vi "Get IP Name.vi"(8 "error in (no error)":errorcluster, 11 "Engine Simulation IP in":refnum<class "Engine Simulation IP.lvclass">) -> (0 "error out":errorcluster, 2 "Name":string, 3 "Engine Simulation IP out":refnum<class "Engine Simulation IP.lvclass">)   [LabVIEW 2013, in "Engine Simulation IP.lvclass"]
uses:
  Engine Simulation IP.lvclass
  Engine Simulation IP.lvclass/Engine Simulation IP.ctl
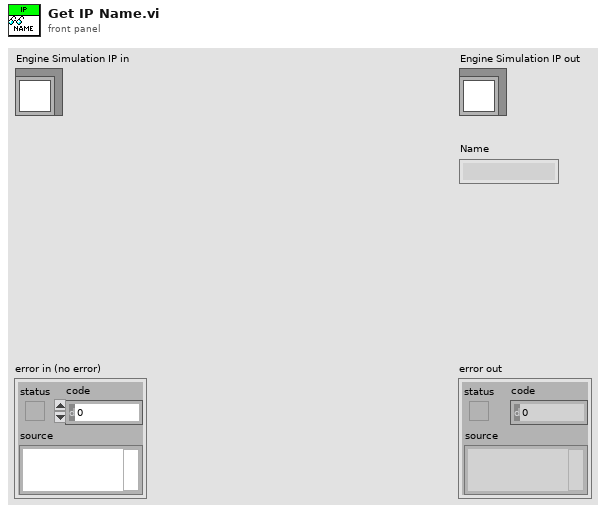
[diagram p1: front panel]
types:
  T1 = typedef "Engine Simulation IP.lvclass/IP class private data.ctl" = cluster{"Name":string, "EST version":T2, "session":refnum<class "Engine Simulation Session.lvclass">}
  T2 = typedef "Engine Simulation Session.lvclass/Bitfile Major Version.ctl" = enum16{"1.0", "1.1", "1.2", "1.3"}
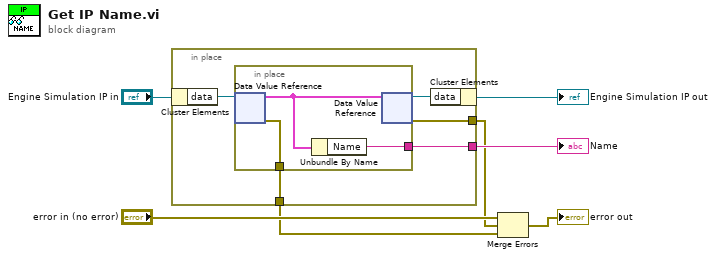
[diagram p0: block diagram]
diagram:
  n1 = in-place {
    in-place-border: [w12] -> w6
    in-place-border: [w9] -> w2
    in-place-border: [w8] -> w1
    n2 = in-place-cluster #1("Engine Simulation IP in") -> ("data"=w11:refnum<data-value>)
    n3 = in-place {
      in-place-border: [w15] -> w12
      in-place-border: [w13] -> w8
      n4 = in-place-dvr #2(w11) -> (w14:T1, w13:errorcluster)
      n5 = Unbundle By Name(w14) -> ("Name"=w15:string)
      n6 = in-place-dvr #2(w14) -> (w10:refnum<data-value>, w9:errorcluster)
    }
    n7 = in-place-cluster #1("data"=w10) -> (→"Engine Simulation IP out":refnum<class "Engine Simulation IP.lvclass">)
  }
  "Name" <- w6
  n8 = Merge Errors("error in (no error)", w2, w1) -> (→"error out":errorcluster)
